vi "setDcOffset.vi"(7 "Channel":string="0", 8 "error in (no error)":errorcluster, 10 "Offset [V]":dbl, 11 "FgenNiPxi in":refnum<class "ArbNi.lvclass">) -> (0 "error out":errorcluster, 3 "FgenNiPxi out":refnum<class "ArbNi.lvclass">)   [LabVIEW 2023, in "ArbNi.lvclass"]
doc: "<b>Author:</b> Wolfgang\n<b>Description:</b> Set DC Offset in V."
uses:
  ArbNi.lvclass
  ArbNi.lvclass/ArbNi.ctl
  Arb.lvclass
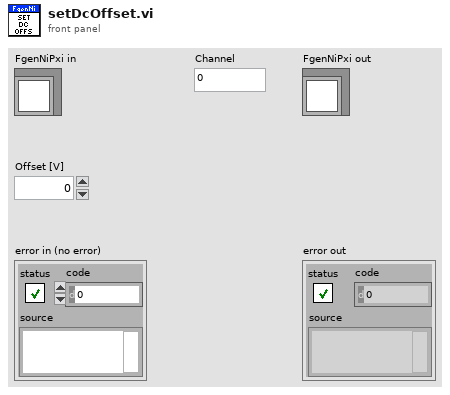
[diagram p1: front panel]
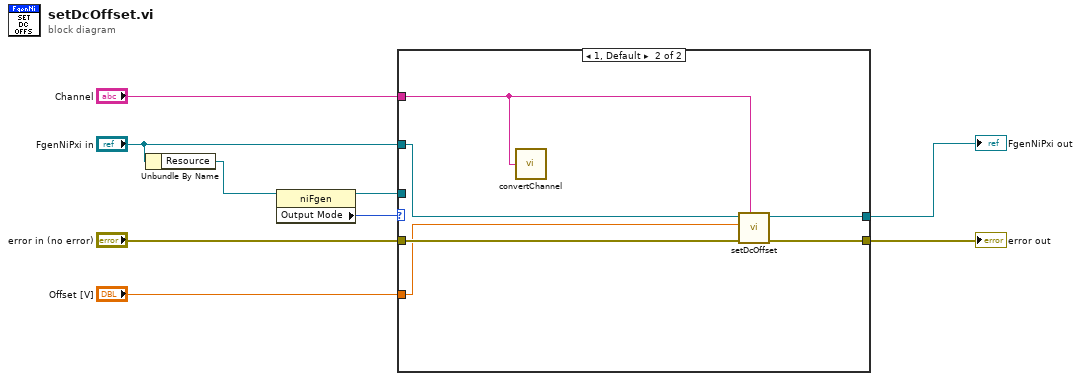
[diagram p0: block diagram]
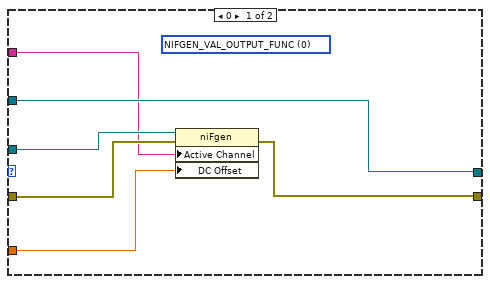
[diagram p2: hidden frame]
diagram:
  n1 = Unbundle By Name("FgenNiPxi in") -> ("Resource"=w1:refnum<k15>)
  n2 = property class="niFgen"(reference=w1) -> (reference out=w2:refnum<k15>, "Output Mode"=w3:i32)  [unwired: 1 in, 1 out]
  n3 = case shown="1, Default" w3 {
    tunnel: [w11 w21] -> w9
    tunnel: [w13 w20] -> w8
    tunnel: "error in (no error)" -> [w12 w19]
    tunnel: "FgenNiPxi in" -> [w13 w18]
    tunnel: "Offset [V]" -> [w14 w17]
    tunnel: "Channel" -> [w10 w16]
    tunnel: w2 -> [w15 _]
    frame 0 {
      (unwired) 0 items=["NIFGEN_VAL_OUTPUT_FUNC"=0, "NIFGEN_VAL_OUTPUT_FREQ_LIST"=101, "NIFGEN_VAL_OUTPUT_ARB"=1, "NIFGEN_VAL_OUTPUT_SEQ"=2, "NIFGEN_VAL_OUTPUT_SCRIPT"=102] ("Output:Output Mode")
      n4 = property class="niFgen"(reference=w15, error in=w12, "Active Channel"=w10, "DC Offset"=w14) -> (error out=w11:errorcluster)  [unwired: 1 out]
    }
    frame 1, Default {
      n5 = call "convertChannel.vi"("Channel"=w16) -> ()  [unwired: 1 out]
      n6 = call-parent "setDcOffset.vi"("Channel"=w16, "error in (no error)"=w19, "Offset [V]"=w17, "Fgen in"=w18) -> ("error out"=w21:errorcluster, "Fgen out"=w20:refnum<class "ArbNi.lvclass">)  [unwired: 6 in]
    }
  }
  "error out" <- w9
  "FgenNiPxi out" <- w8
